vi "Event Structure String 4.vi"() -> ()   [LabVIEW 2020]
panel:
  out "length":i32
  out "OldVal":string
  out "NewVal":string
  in  "String":string
  in  "Stop":bool
  # "Event Structure String"
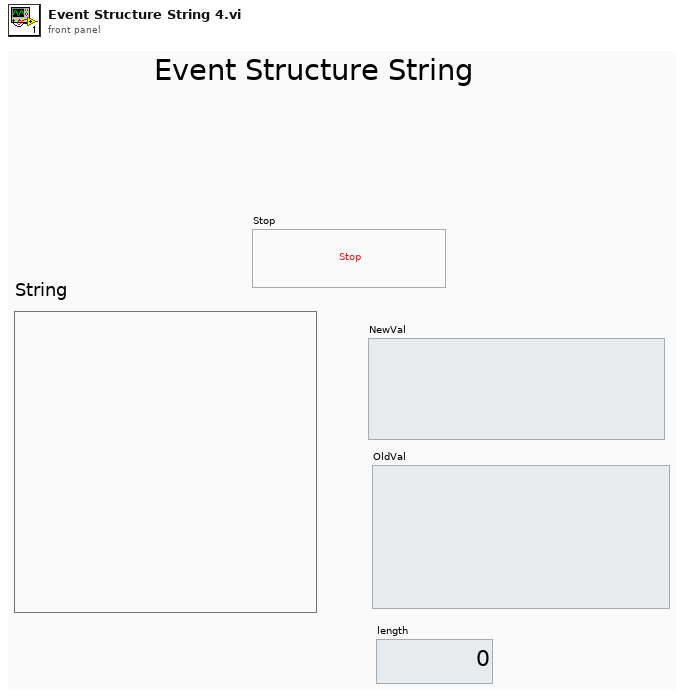
[diagram p1: front panel]
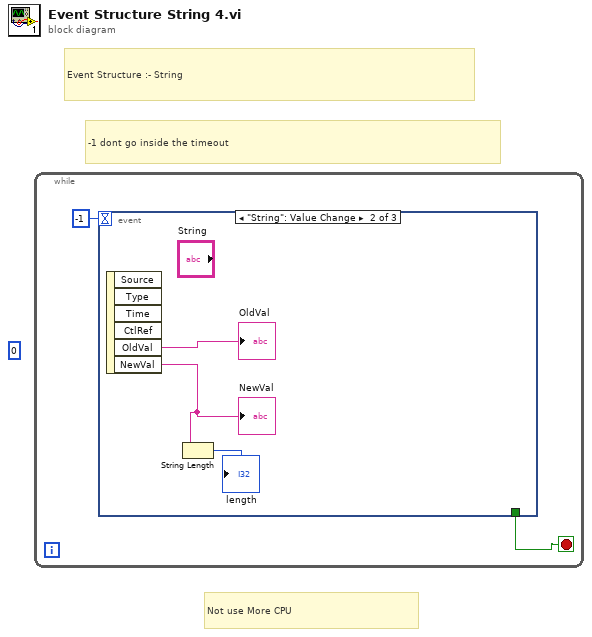
[diagram p0: block diagram]
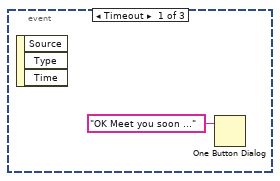
[diagram p2: hidden frame]
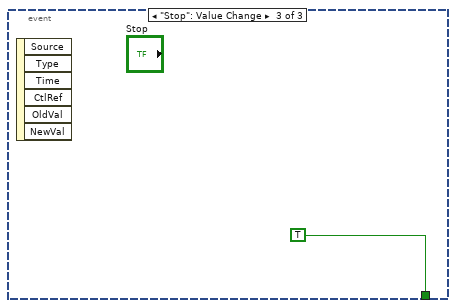
[diagram p3: hidden frame]
diagram:
  (unwired) 0
  # "Not use More CPU"
  # "-1 dont go inside the timeout"
  # "Event Structure :- String"
  n1 = while {
    stop <- w1 stop-if-true
    n2 = event shown="[1] \"String\": Value Change" {
      selector: _ -> [_ _ _]
      dyn-events: _ -> [_ _ _]
      timeout: -1 -> [_ _ _]
      tunnel: [_ _ TRUE] -> w1
      event Timeout {
        n3 = event-data() -> ()  [unwired: 1 in, 3 out]
        n4 = One Button Dialog(message="OK Meet you soon ...") -> ()  [unwired: 1 in, 1 out]
      }
      event "String": Value Change {
        n5 = event-data() -> ("OldVal"=→"OldVal":string, "NewVal"=w5:string)  [unwired: 1 in, 4 out]
        "NewVal" <- w5
        n6 = String Length(string=w5) -> (length=→"length":i32)
      }
      event "Stop": Value Change {
        n7 = event-data() -> ()  [unwired: 1 in, 6 out]
      }
    }
  }
